vi "EnqueueDrive.vi"(8 "error in (no error)":errorcluster, 11 "DriveInstruction":T1) -> (0 "error out":errorcluster)   [LabVIEW 2013]
uses:
  DriveData.ctl
  DriveInstruction.ctl
  QueueSubsystem.ctl
  TankDriveAction.ctl
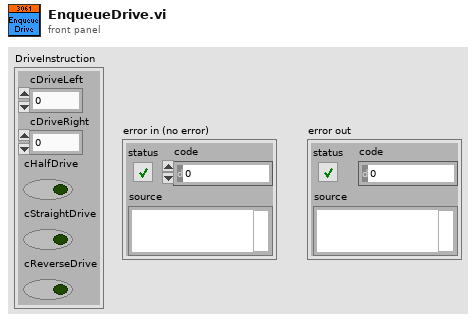
[diagram p1: front panel]
types:
  T1 = typedef "DriveData.ctl" = cluster{"cDriveLeft":dbl, "cDriveRight":dbl, "cHalfDrive":bool, "cStraightDrive":bool, "cReverseDrive":bool}
  T2 = typedef "TankDriveAction.ctl" = enum16{"Init", "LinearDrive", "SetValue", "Disable"}
  T3 = typedef "QueueSubsystem.ctl" = enum16{"Drive", "SonicShifter", "Kicker", "FiringPneumatic", "RollerPneumatic", "Clapper", "RollerMotor", "CollectorMotor", "Servo", "ShooterWrapper", "CollectorWrapper", "CatcherWrapper", "AutoDistance", "PassWrapper"}
  T4 = typedef "DriveInstruction.ctl" = cluster{"DriveData":T1, "Subsystem":T3, "Action":T2}
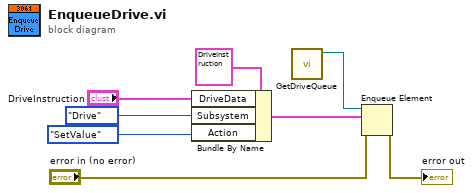
[diagram p0: block diagram]
diagram:
  n1 = Bundle By Name(cluster=T4 {"DriveData"={"cDriveLeft"=0.0, "cDriveRight"=1.0, "cHalfDrive"=FALSE, "cStraightDrive"=FALSE, "cReverseDrive"=FALSE}, "Subsystem"=enum."SonicShifter", "Action"=enum."Init"} ("DriveQueueInstruction"), "DriveData"="DriveInstruction", "Subsystem"=QueueSubsystem."Drive", "Action"=TankDriveAction."SetValue") -> (w3:T4)
  n2 = call "GetDriveQueue.vi"() -> ("queue out"=w6:refnum<queue>)  [unwired: 10 in, 1 out]
  n3 = Enqueue Element(queue=w6, element=w3, error in (no error)="error in (no error)") -> (error out=→"error out":errorcluster)  [unwired: 1 in, 2 out]
